vi "Write Category.vi"(8 "error in (no error)":errorcluster, 10 "Category":enum16{"Public API", "Constant VI", "Error VI"}(ring), 11 "VI in":refnum<class "VI.lvclass">) -> (0 "error out":errorcluster, 3 "VI out":refnum<class "VI.lvclass">)   [LabVIEW 2019, in "VI.lvclass"]
uses:
  VI.lvclass
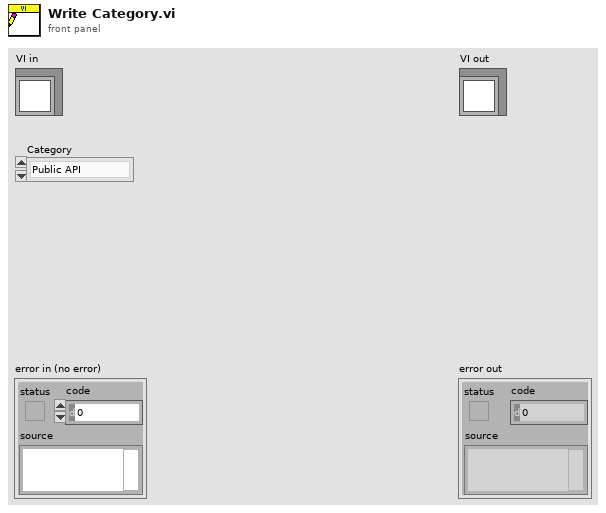
[diagram p1: front panel]
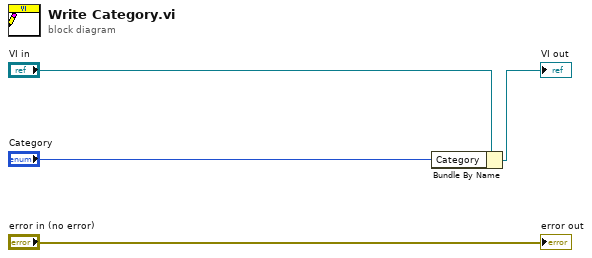
[diagram p0: block diagram]
diagram:
  n1 = Bundle By Name(cluster="VI in", "Category"="Category") -> (→"VI out":refnum<class "VI.lvclass">)
  "error out" <- "error in (no error)"
